vi "2015 Write Summary Data.vi"(7 "2015 Cycle Stats":T1, 8 "Error In":errorcluster, 10 "Write Header?":bool, 11 "new file path (Not A Path if cancelled)":path) -> (0 "Error Out":errorcluster)   [LabVIEW 2014]
uses:
  Type Definitions/2015 Program/2015 Cycle Stats.ctl
  <vilib>/Utility/file.llb/Write To Spreadsheet File (string).vi
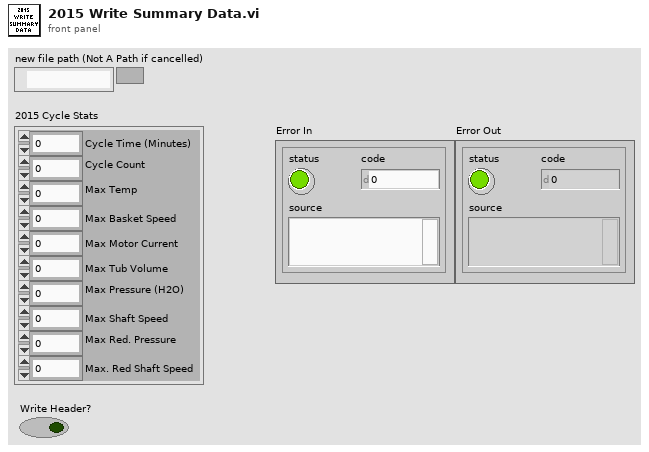
[diagram p1: front panel]
types:
  T1 = typedef "2015 Cycle Stats.ctl" = cluster{"Cycle Time (Minutes)":dbl, "Max Temp":dbl, "Max Basket Speed":dbl, "Max Motor Current":dbl, "Max Tub Volume":dbl, "Max Pressure (H2O)":dbl, "Cycle Count":dbl, "Max Shaft Speed ":dbl, "Max Red. Pressure":dbl, "Max. Red Shaft Speed":dbl}
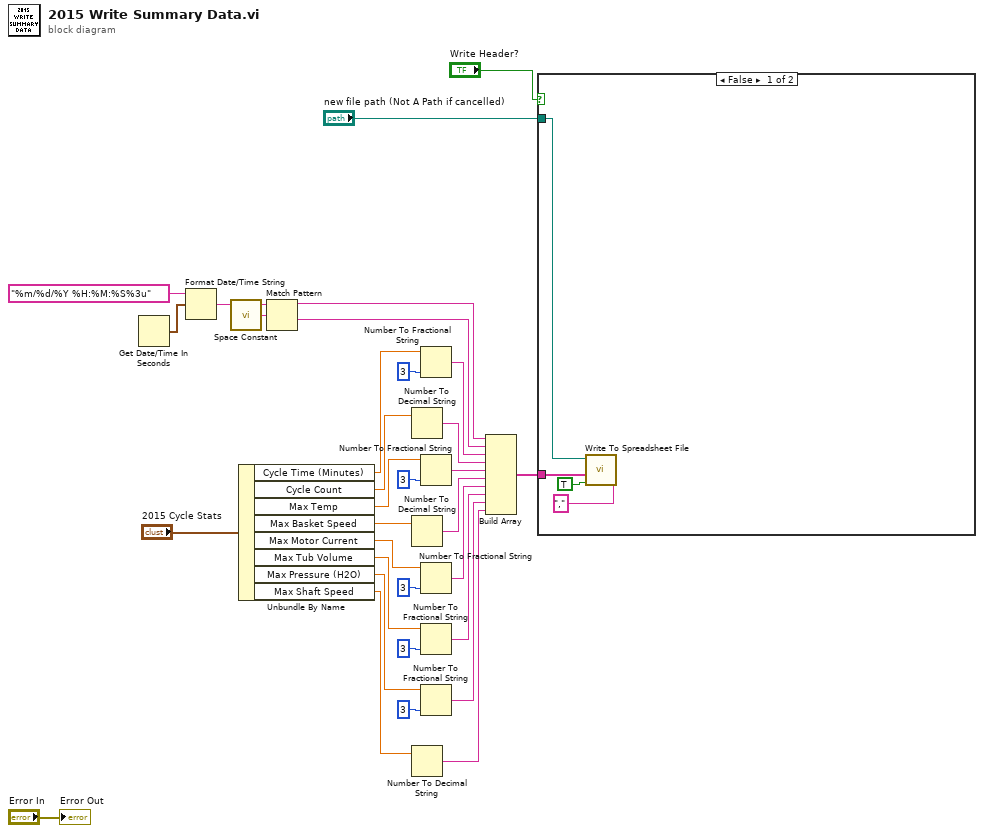
[diagram p0: block diagram]
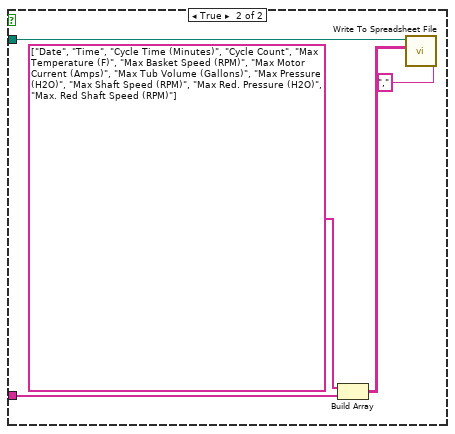
[diagram p2: hidden frame]
diagram:
  n1 = Get Date/Time In Seconds() -> (seconds since 1Jan1904=w5:timestamp)
  n2 = Format Date/Time String(time format string (%c)="%m/%d/%Y %H:%M:%S%3u", seconds (now)=w5) -> (date/time string=w3:string)  [unwired: 1 in]
  n3 = call <vilib>:"Space Constant.vi"() -> ("String"=w2:string)
  n4 = Unbundle By Name("2015 Cycle Stats") -> ("Cycle Time (Minutes)"=w25:dbl, "Cycle Count"=w26:dbl, "Max Temp"=w27:dbl, "Max Basket Speed"=w28:dbl, "Max Motor Current"=w29:dbl, "Max Tub Volume"=w30:dbl, "Max Pressure (H2O)"=w31:dbl, "Max Shaft Speed"=w32:dbl)
  n5 = Match Pattern(string=w3, regular expression=w2) -> (before substring=w9:string, after substring=w10:string)  [unwired: 1 in, 2 out]
  n6 = Number To Decimal String(number=w26) -> (decimal integer string=w13:string)  [unwired: 1 in]
  n7 = Number To Decimal String(number=w28) -> (decimal integer string=w16:string)  [unwired: 1 in]
  n8 = Number To Decimal String(number=w32) -> (decimal integer string=w20:string)  [unwired: 1 in]
  n9 = Number To Fractional String(number=w25, precision (6)=i16 3) -> (F-format string=w12:string)  [unwired: 2 in]
  n10 = Number To Fractional String(number=w27, precision (6)=i16 3) -> (F-format string=w15:string)  [unwired: 2 in]
  n11 = Number To Fractional String(number=w29, precision (6)=i16 3) -> (F-format string=w17:string)  [unwired: 2 in]
  n12 = Number To Fractional String(number=w30, precision (6)=i16 3) -> (F-format string=w18:string)  [unwired: 2 in]
  n13 = Number To Fractional String(number=w31, precision (6)=i16 3) -> (F-format string=w19:string)  [unwired: 2 in]
  n14 = Build Array(w9, w10, w12, w13, w15, w16, w17, w18, w19, w20) -> (w21:string[])
  n15 = case shown="False" "Write Header?" {
    tunnel: w21 -> [w34 w40]
    tunnel: "new file path (Not A Path if cancelled)" -> [w35 w38]
    frame False {
      n16 = call-poly <vilib>:"Write To Spreadsheet File.vi"("delimiter (\\t)"="," ("delimiter (\\t)"), "append to file? (new file:F)"=TRUE, "1D data"=w34, "file path (dialog if empty)"=w35) -> ()  [unwired: 4 in, 1 out]
    }
    frame True {
      n17 = Build Array(string[] ["Date", "Time", "Cycle Time (Minutes)", "Cycle Count", "Max Temperature (F)", "Max Basket Speed (RPM)", "Max Motor Current (Amps)", "Max Tub Volume (Gallons)", "Max Pressure (H2O)", "Max Shaft Speed (RPM)", "Max Red. Pressure (H2O)", "Max. Red Shaft Speed (RPM)"], w40) -> (w37:string[][])
      n18 = call-poly <vilib>:"Write To Spreadsheet File.vi"("delimiter (\\t)"="," ("delimiter (\\t)"), "2D data"=w37, "file path (dialog if empty)"=w38) -> ()  [unwired: 5 in, 1 out]
    }
  }
  "Error Out" <- "Error In"
